vi "Janis_AC_3Channel_LKS331_6SRS830.vi"() -> ()   [LabVIEW 2014]
panel:
  out "PeakToPeak\nPiezoVoltage":dbl format="%#_13g"
  out "TimeStamp":dbl format="%#_13g"
  out "Y6":dbl
  out "X6":dbl
  out "Y5":dbl
  out "X5":dbl
  out "Y4":dbl
  out "X4":dbl
  out "Y3":dbl
  out "X3":dbl
  out "T2":dbl
  out "T1":dbl
  out "Y2":dbl
  out "Y1":dbl
  out "X2":dbl
  out "X1":dbl
  in  "Tab Control":enum32{"Set Up", "R0 Vs T", "dV/dstrain Vs T"}(tab)
  in  "PiezoDrive":refnum<visa-resource-name>
  in  "PiezoGain":dbl
  in  "LKS Temp Controller":refnum<visa-resource-name>
  in  "Sample 2 V0":refnum<visa-resource-name>
  in  "Sample 1 V0":refnum<visa-resource-name>
  in  "SampleName":string
  in  "Sample \nThermometer":enum16{"T1", "T2"}(ring)
  in  "SG dV/dstrain":refnum<visa-resource-name>
  in  "Sample 2 dV/dstrain":refnum<visa-resource-name>
  in  "Sample 1 dV/dstrain":refnum<visa-resource-name>
  in  "SG V0":refnum<visa-resource-name>
  out "XY Graph 6":cluster{dbl, dbl}[](graph) caption="Temp Channel A"
  out "XY Graph 5":cluster{dbl, dbl}[](graph) caption="Temp Channel B"
  out "XY Graph 4":cluster{dbl, dbl}[](graph) caption="SRS1"
  out "XY Graph 4":cluster{dbl, dbl}[](graph) caption="SRS1"
  out "XY Graph 4":cluster{dbl, dbl}[](graph) caption="SRS1"
  out "XY Graph 4":cluster{dbl, dbl}[](graph) caption="SRS1"
  out "XY Graph 4":cluster{dbl, dbl}[](graph) caption="SRS1"
  out "XY Graph 4":cluster{dbl, dbl}[](graph) caption="SRS1"
  out "XY Graph 4":cluster{dbl, dbl}[](graph) caption="SRS1"
  out "XY Graph 4":cluster{dbl, dbl}[](graph) caption="SRS1"
  out "XY Graph 4":cluster{dbl, dbl}[](graph) caption="SRS1"
  out "XY Graph 4":cluster{dbl, dbl}[](graph) caption="SRS1"
  out "XY Graph 4":cluster{dbl, dbl}[](graph) caption="SRS1"
  out "XY Graph 4":cluster{dbl, dbl}[](graph) caption="SRS1"
  out "Data is being stored here":string
  # "RealTime Data"
  # "Thermometry"
  # "INSTRUMENT ADDRESSES"
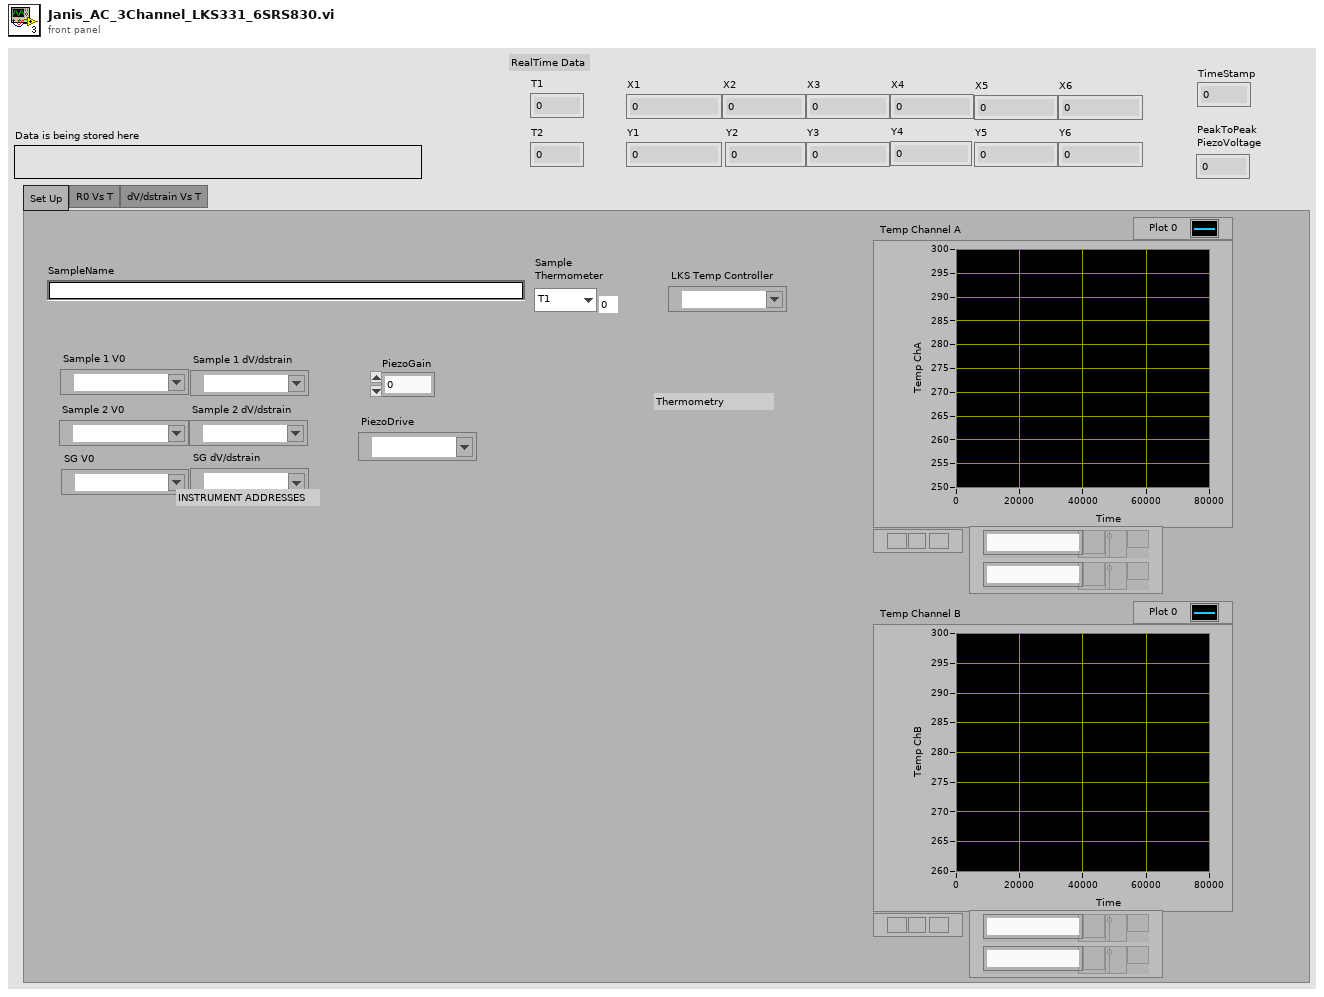
[diagram p1: front panel]
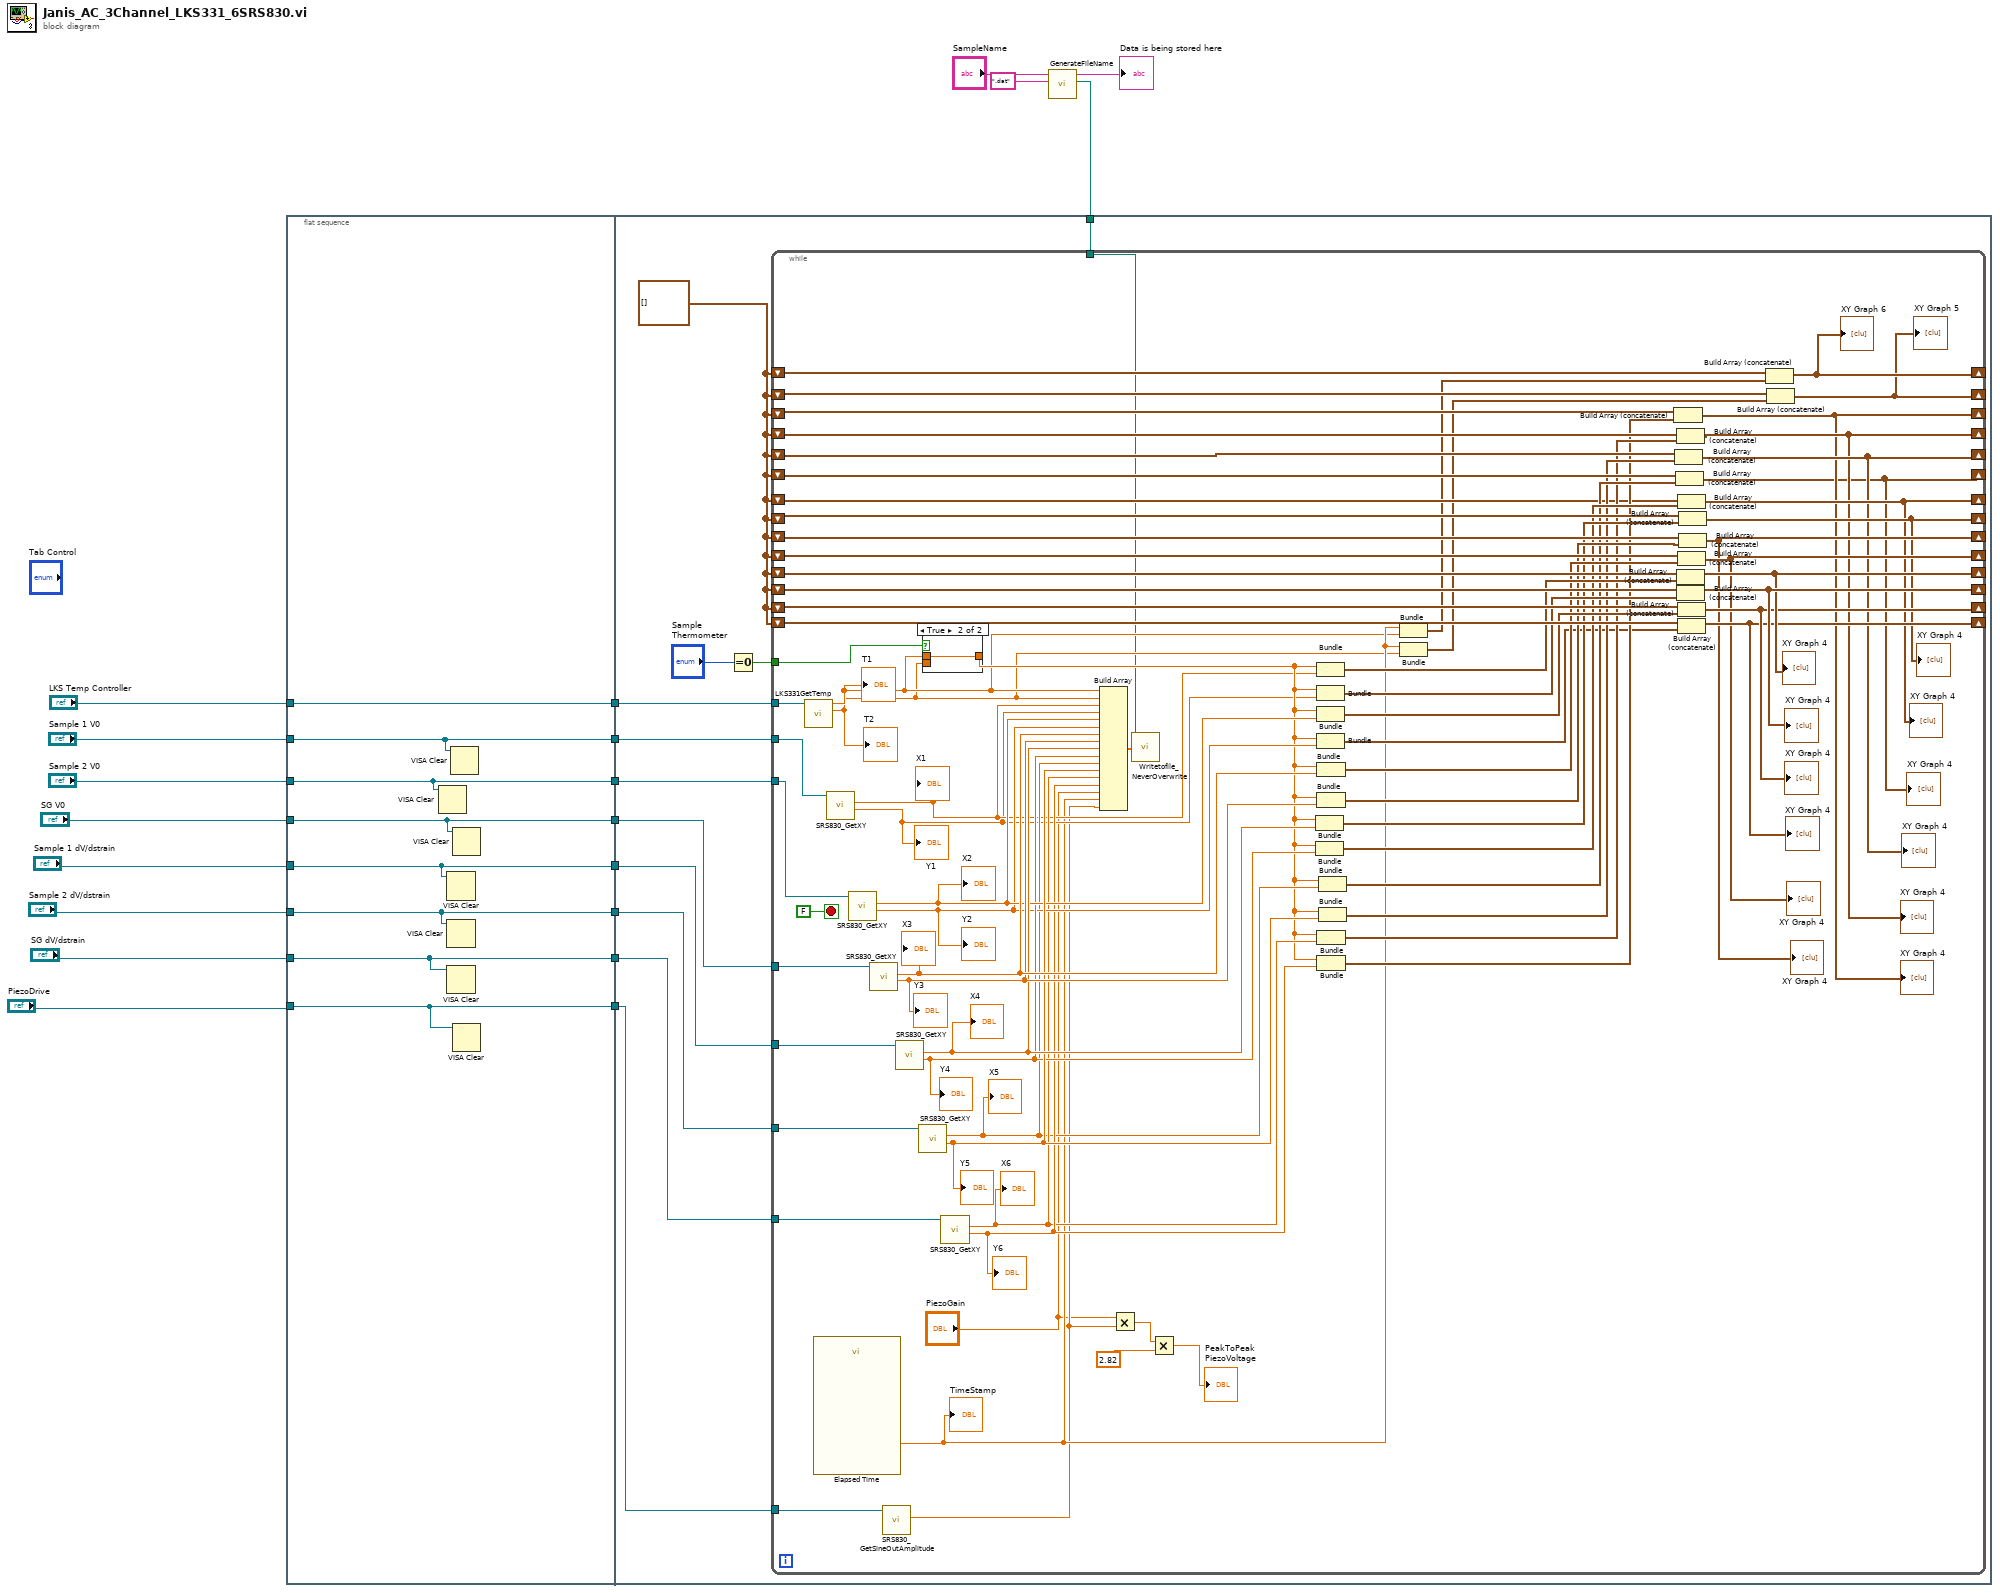
[diagram p0: block diagram]
diagram:
  n1 = flat-sequence {
    tunnel: "Sample 2 V0" -> [w25]
    tunnel: "Sample 1 V0" -> [w26]
    tunnel: "LKS Temp Controller" -> [w28]
    tunnel: [w28] -> w14
    tunnel: [w26] -> w13
    tunnel: [w25] -> w12
    tunnel: "SG V0" -> [w24]
    tunnel: [w24] -> w10
    tunnel: "Sample 1 dV/dstrain" -> [w23]
    tunnel: [w23] -> w9
    tunnel: [w22] -> w8
    tunnel: "Sample 2 dV/dstrain" -> [w22]
    tunnel: [w27] -> w7
    tunnel: "SG dV/dstrain" -> [w27]
    tunnel: "PiezoDrive" -> [w21]
    tunnel: [w21] -> w2
    tunnel: w14 -> [w40]
    tunnel: w13 -> [w39]
    tunnel: w12 -> [w38]
    tunnel: w11 -> [w37]
    tunnel: w10 -> [w34]
    tunnel: w9 -> [w33]
    tunnel: w8 -> [w32]
    tunnel: w7 -> [w31]
    tunnel: w2 -> [w29]
    frame #0 {
      n2 = VISA Clear(VISA resource name=w25) -> ()  [unwired: 1 in, 2 out]
      n3 = VISA Clear(VISA resource name=w23) -> ()  [unwired: 1 in, 2 out]
      n4 = VISA Clear(VISA resource name=w22) -> ()  [unwired: 1 in, 2 out]
      n5 = VISA Clear(VISA resource name=w27) -> ()  [unwired: 1 in, 2 out]
      n6 = VISA Clear(VISA resource name=w26) -> ()  [unwired: 1 in, 2 out]
      n7 = VISA Clear(VISA resource name=w24) -> ()  [unwired: 1 in, 2 out]
      n8 = VISA Clear(VISA resource name=w21) -> ()  [unwired: 1 in, 2 out]
    }
    frame #1 {
      w30 = cluster{"T1":dbl, "Elapsed Time (s)":dbl}[] []
      n9 = Equal To 0?(x="Sample \nThermometer") -> (x = 0?=w36:bool)
      n10 = while {
        tunnel: w40 -> [w114]
        tunnel: w39 -> [w113]
        tunnel: w38 -> [w112]
        tunnel: w37 -> [w42]
        tunnel: w36 -> [w111]
        shift-right: [w97] -> _
        shift-left: w30 -> [w107]
        shift-right: [w96] -> _
        shift-left: w30 -> [w110]
        shift-right: [w99] -> _
        shift-left: w30 -> [w108]
        shift-right: [w98] -> _
        shift-left: w30 -> [w109]
        tunnel: w34 -> [w103]
        tunnel: w33 -> [w102]
        tunnel: w32 -> [w101]
        tunnel: w31 -> [w100]
        shift-right: [w77] -> _
        shift-left: w30 -> [w93]
        shift-right: [w75] -> _
        shift-left: w30 -> [w95]
        shift-right: [w74] -> _
        shift-left: w30 -> [w69]
        shift-right: [w76] -> _
        shift-left: w30 -> [w94]
        shift-right: [w71] -> _
        shift-left: w30 -> [w92]
        shift-right: [w72] -> _
        shift-left: w30 -> [w91]
        shift-right: [w73] -> _
        shift-left: w30 -> [w90]
        shift-right: [w68] -> _
        shift-left: w30 -> [w89]
        shift-right: [w50] -> _
        shift-left: w30 -> [w57]
        shift-right: [w49] -> _
        shift-left: w30 -> [w56]
        tunnel: w29 -> [w48]
        stop <- FALSE stop-if-true
        n11 = call "LKS331GetTemp.vi"("LKS Temp Controller"=w114) -> ("T2"=w53:dbl, "T1"=w54:dbl)  [unwired: 8 in, 1 out]
        "T1" <- w54
        "T2" <- w53
        n12 = call "Elapsed Time"() -> ("Elapsed Time (s)"=w55:dbl)  [unwired: 12 in, 7 out]
        "TimeStamp" <- w55
        n13 = call "SRS830_GetXY.vi"("SRS 830"=w113) -> ("Y"=w58:dbl, "X"=w59:dbl)  [unwired: 7 in, 2 out]
        "X1" <- w59
        "Y1" <- w58
        n14 = call "SRS830_GetXY.vi"("SRS 830"=w112) -> ("Y"=w64:dbl, "X"=w66:dbl)  [unwired: 7 in, 2 out]
        "X2" <- w66
        "Y2" <- w64
        n15 = call "SRS830_GetXY.vi"("SRS 830"=w103) -> ("Y"=w87:dbl, "X"=w88:dbl)  [unwired: 7 in, 2 out]
        "X3" <- w88
        "Y3" <- w87
        n16 = call "SRS830_GetSineOutAmplitude.vi"("VISA resource name"=w48) -> ("Measurement"=w47:dbl)  [unwired: 8 in, 2 out]
        n17 = call "SRS830_GetXY.vi"("SRS 830"=w102) -> ("Y"=w65:dbl, "X"=w81:dbl)  [unwired: 7 in, 2 out]
        "X4" <- w81
        "Y4" <- w65
        n18 = call "SRS830_GetXY.vi"("SRS 830"=w101) -> ("Y"=w67:dbl, "X"=w61:dbl)  [unwired: 7 in, 2 out]
        "X5" <- w61
        "Y5" <- w67
        n19 = case shown="True" w111 {
          tunnel: w54 -> [_ w117]
          tunnel: w53 -> [w116 _]
          tunnel: [w116 w117] -> w60
          frame False {
          }
          frame True {
          }
        }
        n20 = call "SRS830_GetXY.vi"("SRS 830"=w100) -> ("Y"=w63:dbl, "X"=w62:dbl)  [unwired: 7 in, 2 out]
        "X6" <- w62
        "Y6" <- w63
        n21 = Build Array(w54, w53, w59, w58, w66, w64, w88, w87, w81, w65, w61, w67, w62, w63, "PiezoGain", w55, w47) -> (w41:dbl[])
        n22 = Multiply(x="PiezoGain", y=w47) -> (x*y=w45:dbl)
        n23 = call "Writetofile_NeverOverwrite.vi"("appended array"=w41, "FilePathOut"=w42) -> ()  [unwired: 10 in]
        n24 = Multiply(x=w45, y=2.82) -> (x*y=→"PeakToPeak\nPiezoVoltage":dbl)
        n25 = Bundle("T1"=w60, "X"=w81) -> (w84:cluster{"T1":dbl, "X":dbl})  [unwired: 1 in]
        n26 = Bundle("T1"=w60, "Y"=w65) -> (w83:cluster{"T1":dbl, "Y":dbl})  [unwired: 1 in]
        n27 = Bundle("T1"=w60, "X"=w59) -> (w106:cluster{"T1":dbl, "X":dbl})  [unwired: 1 in]
        n28 = Bundle("T1"=w60, "Y"=w58) -> (w105:cluster{"T1":dbl, "Y":dbl})  [unwired: 1 in]
        n29 = Bundle("T1"=w60, "X"=w66) -> (w104:cluster{"T1":dbl, "X":dbl})  [unwired: 1 in]
        n30 = Bundle("T1"=w60, "Y"=w64) -> (w70:cluster{"T1":dbl, "Y":dbl})  [unwired: 1 in]
        n31 = Bundle("T1"=w60, "X"=w88) -> (w86:cluster{"T1":dbl, "X":dbl})  [unwired: 1 in]
        n32 = Bundle("T1"=w60, "Y"=w87) -> (w85:cluster{"T1":dbl, "Y":dbl})  [unwired: 1 in]
        n33 = Bundle("T1"=w60, "X"=w62) -> (w79:cluster{"T1":dbl, "X":dbl})  [unwired: 1 in]
        n34 = Bundle("T1"=w60, "Y"=w63) -> (w78:cluster{"T1":dbl, "Y":dbl})  [unwired: 1 in]
        n35 = Bundle("T1"=w60, "X"=w61) -> (w82:cluster{"T1":dbl, "X":dbl})  [unwired: 1 in]
        n36 = Bundle("T1"=w60, "Y"=w67) -> (w80:cluster{"T1":dbl, "Y":dbl})  [unwired: 1 in]
        n37 = Bundle("Elapsed Time (s)"=w55, "T1"=w54) -> (w51:cluster{"Elapsed Time (s)":dbl, "T1":dbl})  [unwired: 1 in]
        n38 = Bundle("Elapsed Time (s)"=w55, "T2"=w53) -> (w52:cluster{"Elapsed Time (s)":dbl, "T2":dbl})  [unwired: 1 in]
        n39 = Build Array (concatenate)(w92, w78) -> (w71:cluster{"T1":dbl, "Y":dbl}[])
        "XY Graph 4" <- w71
        n40 = Build Array (concatenate)(w90, w80) -> (w73:cluster{"T1":dbl, "Y":dbl}[])
        "XY Graph 4" <- w73
        n41 = Build Array (concatenate)(w89, w82) -> (w68:cluster{"T1":dbl, "X":dbl}[])
        "XY Graph 4" <- w68
        n42 = Build Array (concatenate)(w91, w79) -> (w72:cluster{"T1":dbl, "X":dbl}[])
        "XY Graph 4" <- w72
        n43 = Build Array (concatenate)(w109, w106) -> (w98:cluster{"T1":dbl, "X":dbl}[])
        "XY Graph 4" <- w98
        n44 = Build Array (concatenate)(w108, w105) -> (w99:cluster{"T1":dbl, "Y":dbl}[])
        "XY Graph 4" <- w99
        n45 = Build Array (concatenate)(w69, w83) -> (w74:cluster{"T1":dbl, "Y":dbl}[])
        "XY Graph 4" <- w74
        n46 = Build Array (concatenate)(w93, w86) -> (w77:cluster{"T1":dbl, "X":dbl}[])
        "XY Graph 4" <- w77
        n47 = Build Array (concatenate)(w107, w104) -> (w97:cluster{"T1":dbl, "X":dbl}[])
        "XY Graph 4" <- w97
        n48 = Build Array (concatenate)(w110, w70) -> (w96:cluster{"T1":dbl, "Y":dbl}[])
        "XY Graph 4" <- w96
        n49 = Build Array (concatenate)(w95, w84) -> (w75:cluster{"T1":dbl, "X":dbl}[])
        "XY Graph 4" <- w75
        n50 = Build Array (concatenate)(w94, w85) -> (w76:cluster{"T1":dbl, "Y":dbl}[])
        "XY Graph 4" <- w76
        n51 = Build Array (concatenate)(w57, w51) -> (w50:cluster{"Elapsed Time (s)":dbl, "T1":dbl}[])
        "XY Graph 6" <- w50
        n52 = Build Array (concatenate)(w56, w52) -> (w49:cluster{"Elapsed Time (s)":dbl, "T2":dbl}[])
        "XY Graph 5" <- w49
      }
    }
  }
  n53 = call "GenerateFileName.vi"("FileExtension"=".dat", "SampleName"="SampleName") -> ("FilePathOut"=w11:path, "FolderNameString"=→"Data is being stored here":string)  [unwired: 3 in, 1 out]
